vi "GetSetProgramDataString.vi"(0 "VISA resource name":refnum<visa-resource-name>, 5 "get/set":T1=enum."set", 7 "8800 Program Name":string="test", 9 "Number of Intervals":i16=1 min=1 max=300 step=1, 11 "error in":errorcluster) -> (4 "VISA resource name out":refnum<visa-resource-name>, 6 "Program get number of intervals":string, 15 "error out":errorcluster)   [LabVIEW 2023, in "Thermotron 8800.lvlib"]
doc: "PROG\nCommand name: Send or load program data string\nCommand type: Programming\nDescription: This command sets up the 8800 or host computer to load an entire program into the 8800’s program memory. The query command receives the data string from the 8800, while the operation command sends the data string to the 8800. For additional\ninformation, see “Using the interface command set” later in this section.\nThe query command sets up which program will be retrieved, and responds with the\nname of the program and the number of intervals in the program. The operation\ncommand sets up the name and the number of intervals in the program.\nSyntax: PROGname? or PROGn? or PROG, name, number of intervals\nWhere:\nname = program name\nnumber of intervals = integer (1 to 300)\nData type: See Syntax.\nQuery example: PROGtemp_test?\n8800 response: temp_test,6 (The program named “temp_test” is 6 intervals long.)\nOperation example: PROG,HI HUMIDITY,25\n8800 response: 0 (The 8800 will load a 25-interval program and name the program HI HUMIDITY.)"
uses:
  Thermotron 8800.lvlib
  Private/get set.ctl
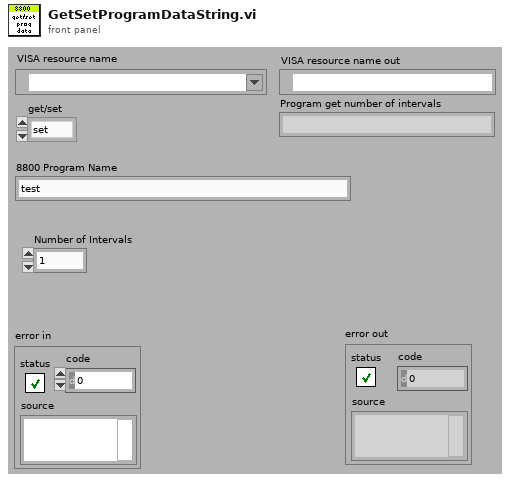
[diagram p1: front panel]
types:
  T1 = typedef "Thermotron 8800.lvlib/get set.ctl" = enum16{"get", "set"}
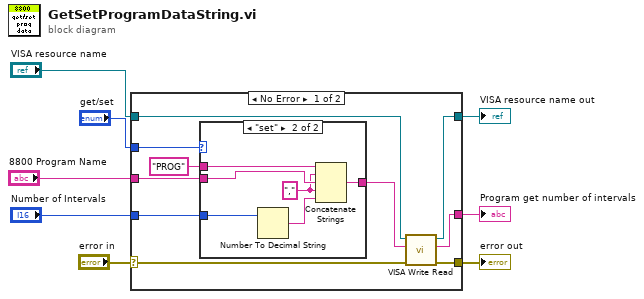
[diagram p0: block diagram]
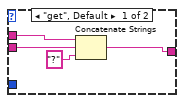
[diagram p2: hidden frame]
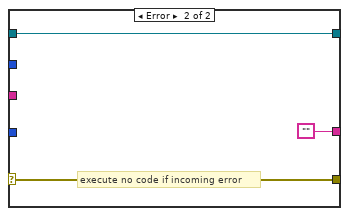
[diagram p3: hidden frame]
diagram:
  n1 = case shown="No Error" "error in" {
    selector: "error in" -> [w17 w31]
    tunnel: [w15 w31] -> w6
    tunnel: [w16 w29] -> w4
    tunnel: "get/set" -> [w13 _]
    tunnel: [w14 ""] -> w3
    tunnel: "VISA resource name" -> [w12 w29]
    tunnel: "8800 Program Name" -> [w10 _]
    tunnel: "Number of Intervals" -> [w9 _]
    frame No Error {
      n2 = case shown="\"set\"" w13 {
        tunnel: [w22 w28] -> w18
        tunnel: "PROG" ("8800 Command") -> [w20 w27]
        tunnel: w10 -> [w19 w26]
        tunnel: w9 -> [_ w24]
        frame "get", Default {
          n3 = Concatenate Strings(w20, w19, "?" ("8800 Command")) -> (w22:string)
        }
        frame "set" {
          w25 = "," ("string")
          n4 = Number To Decimal String(number=w24) -> (decimal integer string=w23:string)  [unwired: 1 in]
          n5 = Concatenate Strings(w27, w25, w26, w25, w23) -> (w28:string)
        }
      }
      n6 = call "VISA Write Read.vi"("error in (no error)"=w17, "8800 Command"=w18, "VISA Refnum in"=w12) -> ("error out"=w15:errorcluster, "read buffer"=w14:string, "VISA Refnum out"=w16:refnum<visa-resource-name>)  [unwired: 6 in]
    }
    frame Error {
      # "execute no code if incoming error"
    }
  }
  "VISA resource name out" <- w4
  "error out" <- w6
  "Program get number of intervals" <- w3
